vi "G4BaseTemplate_Singleton_6x8x6_ReadAttribute.vi"(5 "error in (no error)":errorcluster) -> (19 "error out":errorcluster)   [LabVIEW 2014]
uses:
  <resource>/Framework/Providers/Open_GDS/ClassProviders/Provider_EndevoGOOP400/Templates/G4BaseTemplate_Singleton_6x8x6/G4BaseTemplate_Singleton_6x8x6.lvclass
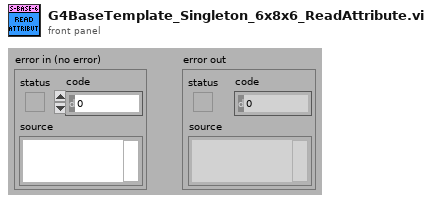
[diagram p1: front panel]
types:
  T1 = typedef "G4BaseTemplate_Singleton_6x8x6.lvclass/ObjectAttributes.ctl" = cluster{"Attribute1":dbl}
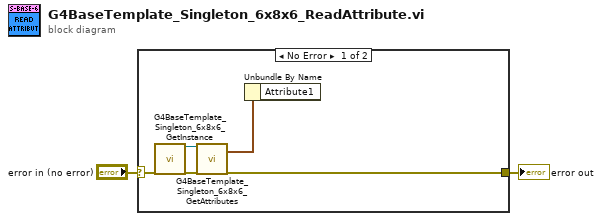
[diagram p0: block diagram]
diagram:
  n1 = case shown="No Error" "error in (no error)" {
    selector: "error in (no error)" -> [w4 w8]
    tunnel: [w6 w8] -> w1
    frame No Error {
      n2 = call <resource>:"G4BaseTemplate_Singleton_6x8x6_GetInstance.vi"("error in (no error)"=w4) -> ("reference out"=w5:refnum<class "G4BaseTemplate_Singleton_6x8x6.lvclass">, "error out"=w3:errorcluster)  [unwired: 14 in, 3 out]
      n3 = call <resource>:"G4BaseTemplate_Singleton_6x8x6_GetAttributes.vi"("reference in"=w5, "error in (no error)"=w3) -> ("Data"=w7:T1, "error out"=w6:errorcluster)  [unwired: 14 in, 2 out]
      n4 = Unbundle By Name(w7) -> ()  [unwired: 1 out]
    }
    frame Error {
    }
  }
  "error out" <- w1
